vi "Plotter_competition - blank subVI.vi"(0 "Switch A Latched":bool=TRUE, 1 "Array":i32[][](array[numeric]), 5 "dt in sec":dbl, 7 "Potentiometer bias (-1 to +1)":dbl, 9 "Encoder 1 count":i64, 11 "Encoder 2 count":i64, 12 "Motor steps 1":i64, 13 "Motor steps 2":i64, 14 "Elapsed Time Out (S)":dbl) -> (4 "Stop":bool, 6 "Motor 1 command":i8=-1, 8 "Motor 2 command":i8=1, 10 "MS lines":bool[](array[boolean]))   [LabVIEW 2014]
panel:
  out "Y Integer to be added/subtracted 2":dbl
  out "X Integer to be added/subtracted":dbl
  out "X0":i32
  out "Y0":i32
  out "X1":i32
  out "Y1":i32
  # "Outputs"
  # "Inputs"
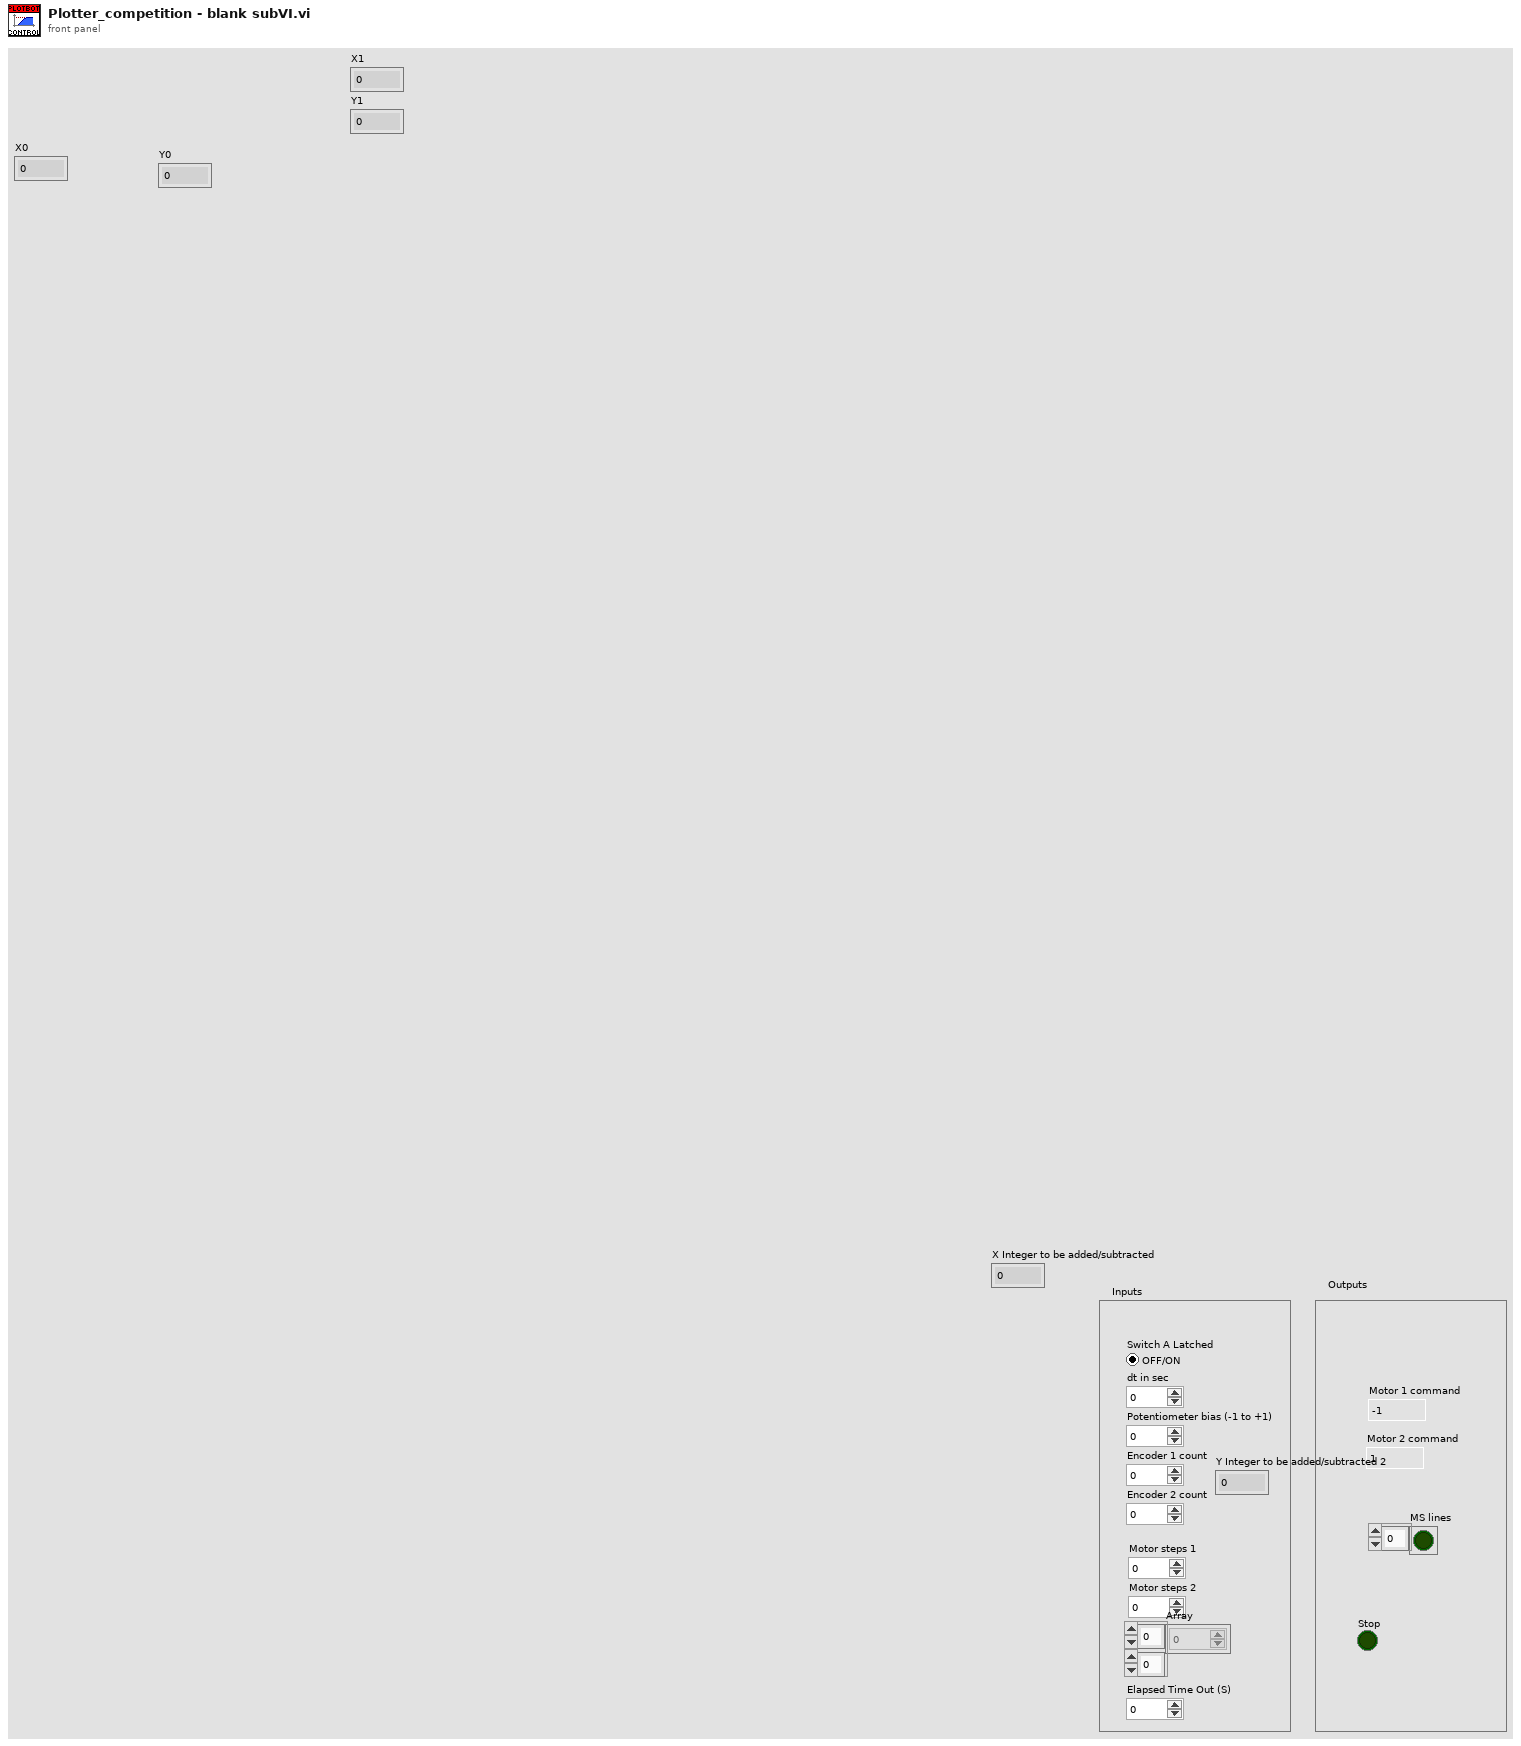
[diagram p1: front panel]
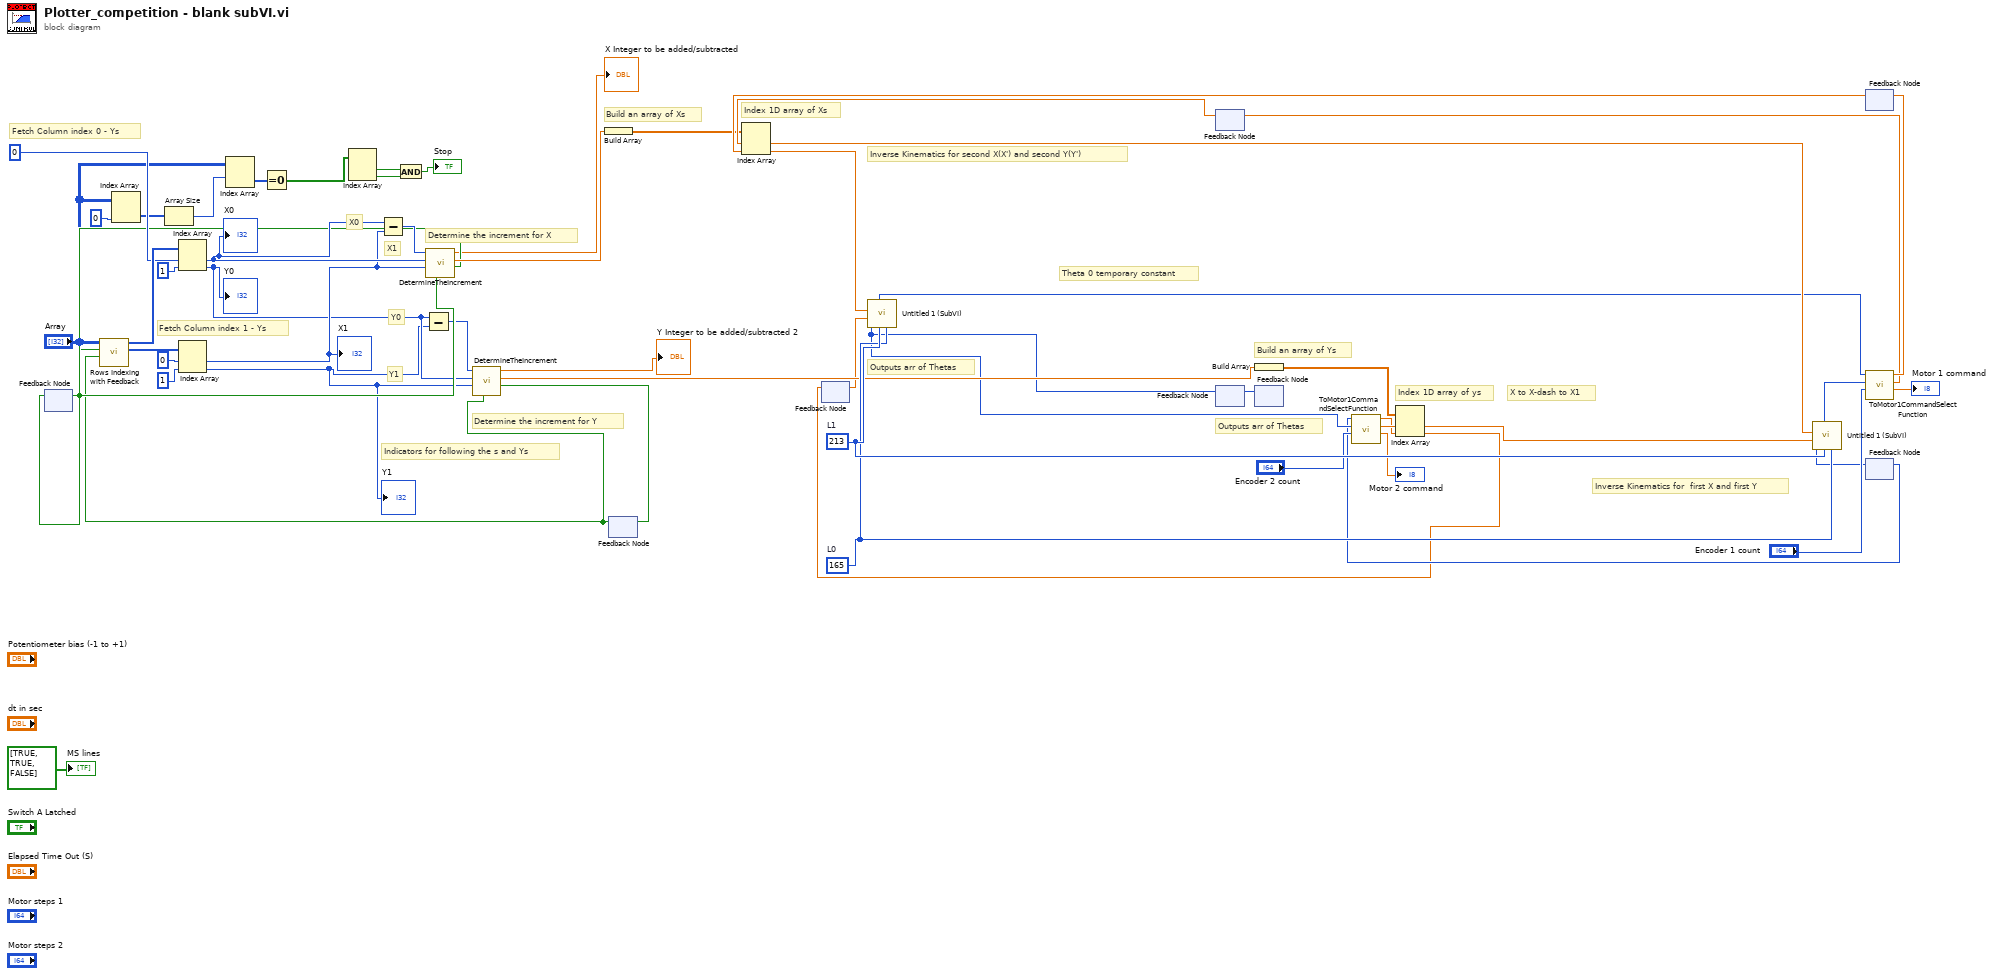
[diagram p0: block diagram]
diagram:
  w48 = 165  # L0
  w49 = 213  # L1
  # "Build an array of Ys"
  # "Index 1D array of ys"
  # "Determine the increment for Y"
  # "X1"
  # "X0"
  # "Y1"
  # "Y0"
  # "Determine the increment for X"
  # "Theta 0 temporary constant"
  # "Fetch Column index 1 - Ys"
  # "Fetch Column index 0 - Ys"
  # "Build an array of Xs"
  # "Outputs arr of Thetas"
  # "Outputs arr of Thetas"
  # "Inverse Kinematics for second X(X') and second Y(Y')"
  # "X to X-dash to X1"
  # "Inverse Kinematics for  first X and first Y"
  # "Index 1D array of Xs"
  # "Indicators for following the s and Ys"
  n1 = feedback #1() -> (w42:bool)  [unwired: 1 in]
  n2 = Index Array(array="Array", index (col)=0 ("disabled index (col)")) -> (element=w15:i32[])  [unwired: 1 in]
  n3 = Array Size(array=w15) -> (size(s)=w8:i32)
  n4 = Index Array(array="Array", index (row)=w8) -> (element=w6:i32[])  [unwired: 1 in]
  n5 = Equal To 0?(x=w6) -> (x = 0?=w4:bool[])
  n6 = Index Array(array=w4) -> (element #1=w3:bool, element #2=w2:bool)  [unwired: 2 in]
  n7 = And(x=w3, y=w2) -> (x .and. y?=→"Stop":bool)
  n8 = feedback #2() -> (w12:bool)  [unwired: 1 in]
  n9 = call "Rows Indexing with Feedback.vi"("Boolean 2"=w12, "Boolean"=w42, "Array 3"="Array") -> ("Array"=w54:i32[], "Array 2"=w55:i32[])  [unwired: 7 in]
  n10 = Index Array(array=w55, index #1=0 ("index"), index #2=1 ("index")) -> (element #1=w53:i32, element #2=w37:i32)
  "X0" <- w53
  "Y0" <- w37
  n11 = Index Array(array=w54, index #1=0 ("index"), index #2=1 ("index")) -> (element #1=w52:i32, element #2=w36:i32)
  "X1" <- w52
  "Y1" <- w36
  n12 = Subtract(x=w53, y=w52) -> (x-y=w51:i32)
  n13 = Subtract(x=w37, y=w36) -> (x-y=w38:i32)
  n14 = call "DetermineTheIncrement.vi"("Boolean in"=w42, "Numeric 3"=w52, "Numeric 4"=w53, "Numeric in"=w51) -> ("Boolean out"=w43:bool, "Numeric out"=w50:dbl, "Integer to be added/subtracted"=→"X Integer to be added/subtracted":dbl)  [unwired: 5 in]
  n15 = feedback-in #1(w43) -> ()
  n16 = call "DetermineTheIncrement.vi"("Boolean in"=w12, "Numeric 3"=w36, "Numeric 4"=w37, "Numeric in"=w38) -> ("Boolean out"=w13:bool, "Numeric out"=w34:dbl, "Integer to be added/subtracted"=→"Y Integer to be added/subtracted 2":dbl)  [unwired: 5 in]
  n17 = Build Array(w50) -> (w14:dbl[])
  n18 = feedback-in #2(w13) -> ()
  n19 = feedback #3() -> (w10:dbl)  [unwired: 1 in]
  n20 = feedback #4() -> (w24:dbl)  [unwired: 1 in]
  n21 = feedback #5() -> (w31:i32)  [unwired: 1 in]
  n22 = Build Array(w34) -> (w33:dbl[])
  n23 = feedback-in #6(w31) -> ()
  n24 = feedback #6() -> ()  [unwired: 2 in]
  n25 = feedback #7() -> (w26:dbl)  [unwired: 1 in]
  n26 = Index Array(array=w14, index #1=w24, index #2=w26) -> (element #1=w30:dbl, element #2=w9:dbl)
  n27 = call "Untitled 1 (SubVI).vi"("L0"=w48, "L1"=w49, "Y1"=w10, "X1"=w9) -> ("theta 0"=w28:i32, "theta 1"=w19:i32)  [unwired: 6 in]
  n28 = feedback-in #5(w19) -> ()
  n29 = feedback #8() -> (w17:i32)  [unwired: 1 in]
  n30 = call "ToMotor1CommandSelectFunction.vi"("Encoder 1 count"="Encoder 2 count", "theta 0"=w19, "theta 1"=w17) -> ("t"=→"Motor 2 command":dbl, "Numeric 2"=w23:dbl, "Numeric"=w22:dbl)  [unwired: 6 in]
  n31 = Index Array(array=w33, index #1=w23, index #2=w22) -> (element #1=w21:dbl, element #2=w11:dbl)
  n32 = feedback-in #3(w11) -> ()
  n33 = call "Untitled 1 (SubVI).vi"("L0"=w48, "L1"=w49, "Y1"=w21, "X1"=w30) -> ("theta 0"=w29:i32, "theta 1"=w18:i32)  [unwired: 6 in]
  n34 = call "ToMotor1CommandSelectFunction.vi"("Encoder 1 count"="Encoder 1 count", "theta 0"=w29, "theta 1"=w28) -> ("t"=→"Motor 1 command":dbl, "Numeric 2"=w25:dbl, "Numeric"=w27:dbl)  [unwired: 6 in]
  n35 = feedback-in #4(w25) -> ()
  n36 = feedback-in #7(w27) -> ()
  n37 = feedback-in #8(w18) -> ()
  "MS lines" <- bool[] [TRUE, TRUE, FALSE] ("MS lines")
